vi "Load Config.vi"(8 "error in (no error)":errorcluster, 11 "Messaging Server Module in":refnum<class "Messaging Server Module.lvclass">) -> (0 "error out":errorcluster, 3 "Messaging Server Module out":refnum<class "Messaging Server Module.lvclass">)   [LabVIEW 2020, in "Volatus.lvlib" / "Messaging Server Module.lvclass"]
uses:
  Messaging Server Module.lvclass
  Messaging Server Module.lvclass/Messaging Server Module.ctl
  Module/Module.lvclass
  VolatusConfig/VolatusConfigElement/VolatusConfigElement.lvclass
  VolatusConfig/VolatusConfig.lvlib
  VolatusConfig/Meta Type.ctl
  VolatusConfig/Cluster/Cluster Config.lvclass
  lv-vecto/Vecto/IP Resolver/IP Resolver.lvclass
  C:/dev/lv20CE/relink/lv-volatus/Volatus/Module/Module.lvclass
  C:/dev/lv20CE/relink/lv-volatus/Volatus/Messaging Server Module/Messaging Server Module.lvclass
  VolatusConfig/Task/Task Config.lvclass
  C:/dev/lv20CE/relink/lv-volatus/VolatusConfig/VolatusConfigElement/VolatusConfigElement.lvclass
  C:/dev/lv20CE/relink/lv-volatus/VolatusConfig/Task/Task Config.lvclass
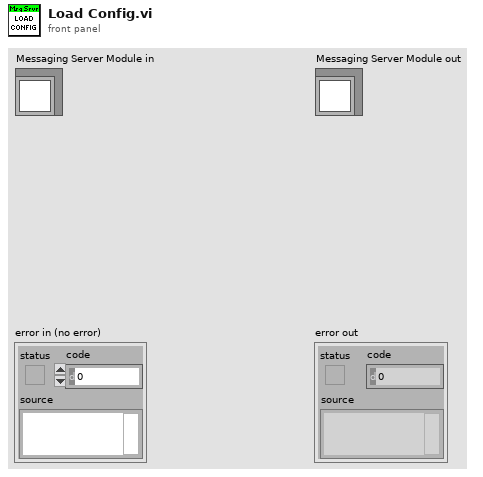
[diagram p1: front panel]
types:
  T1 = typedef "VolatusConfig.lvlib/Meta Type.ctl" = enum16{"UNKNOWN", "VL_System", "VL_Cluster", "VL_Node", "VL_Task", "VL_Group", "VL_Channel", "VL_Task_List", "VL_Scaling", "VL_Sensor", "VL_Sensor_List", "VL_Scale"}
  T2 = typedef "VolatusConfig.lvlib/Messaging Config.ctl" = cluster{"Endpoint":T3, "Allowed Clients":string[]}
  T3 = typedef "VectoConfig.lvlib/Endpoint.ctl" = cluster{"Address":string, "Port":u16}
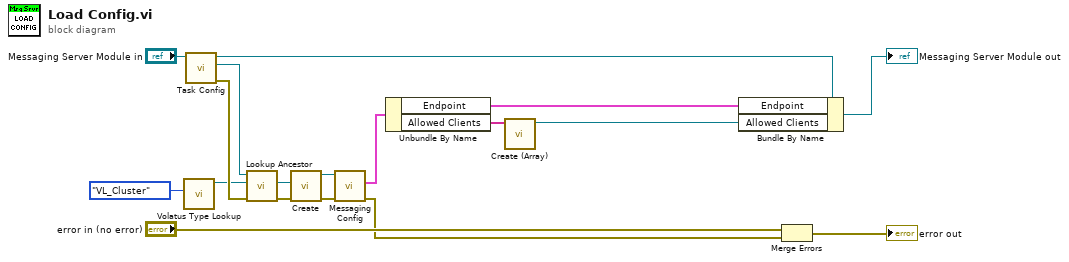
[diagram p0: block diagram]
diagram:
  n1 = call "Volatus Type Lookup.vi"("Meta Type"=Meta_Type."VL_Cluster") -> ("Config Lookup out"=w15:refnum<class "Config Lookup.lvclass">)  [unwired: 9 in, 1 out]
  n2 = call "Task Config.vi"("Module in"="Messaging Server Module in") -> ("error out"=w18:errorcluster, "Task Config"=w4:refnum<class "Task Config.lvclass">, "Module out"=w16:refnum<class "Messaging Server Module.lvclass">)  [unwired: 8 in]
  n3 = call "Lookup Ancestor.vi"("error in (no error)"=w18, "Lookup"=w15, "VolatusConfigElement in"=w4) -> ("error out"=w10:errorcluster, "Ancestor"=w13:refnum<class "Config Element.lvclass">)  [unwired: 6 in, 1 out]
  n4 = call "Create.vi"("error in (no error)"=w10, "Element"=w13) -> ("error out"=w11:errorcluster, "Cluster out"=w12:refnum<class "Cluster Config.lvclass">)  [unwired: 8 in]
  n5 = call "Messaging Config.vi"("error in (no error)"=w11, "Cluster Config in"=w12) -> ("error out"=w1:errorcluster, "Messaging Config"=w9:T2)  [unwired: 7 in, 1 out]
  n6 = Unbundle By Name(w9) -> ("Endpoint"=w7:T3, "Allowed Clients"=w3:string[])
  n7 = call "Create (Array).vi"("Bindings"=w3) -> ("IP Resolver"=w2:refnum<class "IP Resolver.lvclass">)  [unwired: 9 in, 1 out]
  n8 = Bundle By Name(cluster=w16, "Endpoint"=w7, "Allowed Clients"=w2) -> (→"Messaging Server Module out":refnum<class "Messaging Server Module.lvclass">)
  n9 = Merge Errors("error in (no error)", w1) -> (→"error out":errorcluster)
